vi "Do.vi"(8 "error in (no error)":errorcluster, 10 "Actor in":refnum<class "Actor.lvclass">, 11 "Update Array Msg":refnum<class "Update Array Event Msg.lvclass">) -> (0 "error out":errorcluster, 2 "Actor out":refnum<class "Actor.lvclass">)   [LabVIEW 2016, in "Example View Actor.lvlib" / "Update Array Event Msg.lvclass"]
doc: "This VI delivers the message to the actor by calling the appropriate method(s) on the actor."
uses:
  Update Array Event Msg.lvclass
  C:/Project/Shared Libraries/Event Actors/Event Handlers/Abstract Event Message for View/Abstract Event Message for View.lvclass
  <vilib>/ActorFramework/Actor/Actor.lvclass
  Example View Actor/Example View Actor.lvclass
  C:/Program Files (x86)/National Instruments/LabVIEW 2016/vi.lib/ActorFramework/Actor/Actor.lvclass
  Example Events/Double Array Event.lvclass
  Event Handlers/Abstract Event Message for View/Abstract Event Message for View.lvclass/Abstract Event Message for View.ctl
  Example Events/Double Array Event.lvclass/Double Array Event.ctl
  Event Handlers/Abstract Event Message for View/Abstract Event Message for View.lvclass
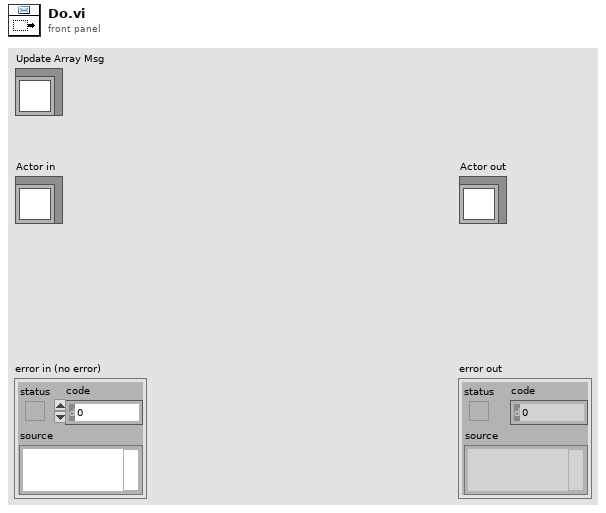
[diagram p1: front panel]
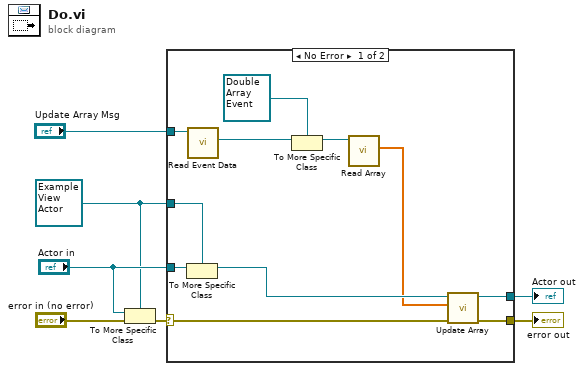
[diagram p0: block diagram]
diagram:
  w2 = refnum<class "Example View Actor.lvclass"> refnum ("Actor in")
  n1 = To More Specific Class(target class=w2, reference="Actor in", error in="error in (no error)") -> (error out=w1:errorcluster)  [unwired: 1 out]
  n2 = case shown="No Error" w1 {
    selector: w1 -> [w16 w20]
    tunnel: [w18 w20] -> w7
    tunnel: [w17 w19] -> w6
    tunnel: "Actor in" -> [w15 w19]
    tunnel: w2 -> [w14 _]
    tunnel: "Update Array Msg" -> [w9 _]
    frame No Error {
      n3 = To More Specific Class(target class=w14, reference=w15) -> (specific class reference=w13:refnum<class "Example View Actor.lvclass">)  [unwired: 1 in, 1 out]
      n4 = call "Read Event Data.vi"("Event Generated Msg"=w9) -> ("Event Data"=w8:refnum<class "Event.lvclass">)  [unwired: 10 in]
      n5 = To More Specific Class(target class=refnum<class "Double Array Event.lvclass"> refnum ("Example Source.lvlib:Double Array Event.lvclass"), reference=w8) -> (specific class reference=w11:refnum<class "Double Array Event.lvclass">)  [unwired: 1 in, 1 out]
      n6 = call "Read Array.vi"("Double Array Event in"=w11) -> ("Array"=w10:dbl[])  [unwired: 9 in, 1 out]
      n7 = call "Update Array.vi"("error in (no error)"=w16, "Array"=w10, "Example Sink In"=w13) -> ("error out"=w18:errorcluster, "Example Sink Out"=w17:refnum<class "Example View Actor.lvclass">)  [unwired: 7 in]
    }
    frame Error {
      # "If type check fails, pass the original object out again."
    }
  }
  "error out" <- w7
  "Actor out" <- w6
